vi "InitGen.vi"(4 "Offset":dbl format="%.4f", 5 "Gain":dbl=1.0 format="%.4f", 6 "Ext/nViTrig":bool, 7 "Waveform Data Array":dbl[](array[numeric]) format="%.4f", 8 "error in (no error)":errorcluster, 9 "Wave Per Pixel":i32, 10 "Sample Rate (Samp/s)":dbl=40000000.0 format="%.2f", 11 "FGEN Resource Name":refnum<k15>) -> (0 "error out":errorcluster, 2 "Actual Sample Rate":dbl, 3 "reference out":refnum<k15>)   [LabVIEW 2020]
uses:
  <instrlib>/niFgen/niFgen.llb/niFgen Output Mode.ctl
  <instrlib>/niFgen/niFgen.llb/niFgen_ctl Sample Clock Source Values (Ring).ctl
  <instrlib>/niFgen/niFgen.llb/niFgen Trigger Mode.ctl
  <instrlib>/niFgen/niFgen.llb/niFgen_ctl Trigger Source Values (Ring).ctl
  <instrlib>/niFgen/niFgen.llb/niFgen_ctl Exported Signal Desination Values (ComboBox).ctl
  <instrlib>/niFgen/niFgen.llb/niFgen_ctl Exported Signal Name Values (Ring).ctl
  <instrlib>/niFgen/niFgen.llb/niFgen Create Waveform (DBL).vi
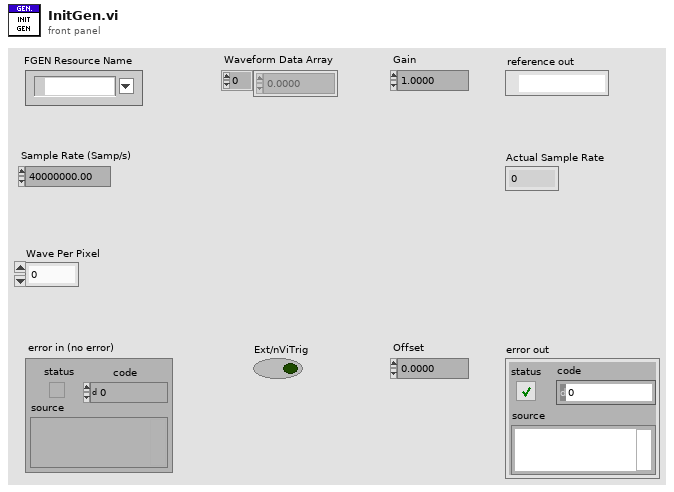
[diagram p1: front panel]
types:
  T1 = typedef "niFgen_ctl Exported Signal Name Values (Ring).ctl" = u16
  T2 = typedef "niFgen_ctl Exported Signal Desination Values (ComboBox).ctl" = string
  T3 = typedef "niFgen_ctl Trigger Source Values (Ring).ctl" = string
  T4 = typedef "niFgen Trigger Mode.ctl" = i32
  T5 = typedef "niFgen_ctl Sample Clock Source Values (Ring).ctl" = string
  T6 = typedef "niFgen Output Mode.ctl" = u32
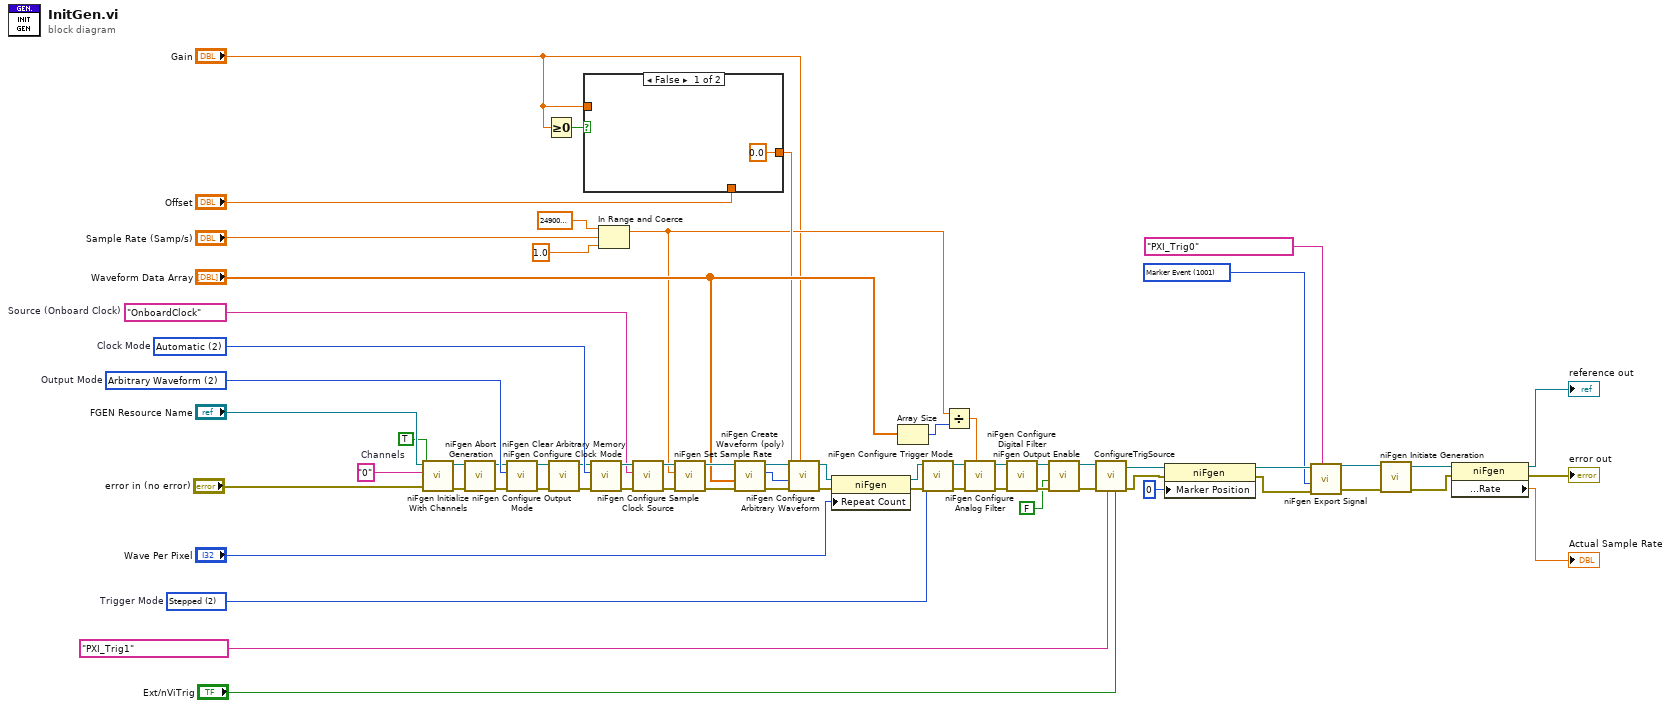
[diagram p0: block diagram]
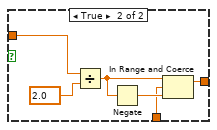
[diagram p2: hidden frame]
diagram:
  w1 = T1 1001 items=["Sample Clock"=101, "Sample Clock Timebase"=1006, "Reference Clock"=102, "Onboard Reference Clock"=1019, "Start Trigger"=1004, "Script Trigger"=103, "Marker Event"=1001, "Data Marker Event"=108, "Ready For Start Event"=105, "Started Event"=106, "Done Event"=107, "Synchronization Pulse"=1007, "Sync Out"=1002] ("Signal")
  w30 = T4 2 items=["Single", "Continuous", "Stepped", "Burst"]  # Trigger Mode
  w50 = T5 "OnboardClock"  # Source (Onboard Clock)
  w64 = u32 2 items=["Hi Resolution Sampling", "Divide Down Sampling", "Automatic"]  # Clock Mode
  w59 = T6 2 items=["Standard Function", "Frequency List", "Arbitrary Waveform", "Arbitrary Sequence", "Script"]  # Output Mode
  w66 = "0"  # Channels
  n1 = call <instrlib>:"niFgen Initialize With Channels.vi"("error in (no error)"="error in (no error)", "Reset Device (default: True)"=TRUE, "Channel Name"=w66, "Resource Name"="FGEN Resource Name") -> ("error out"=w55:errorcluster, "Instrument Handle Out"=w56:refnum<k15>)  [unwired: 6 in]
  n2 = call <instrlib>:"niFgen Abort Generation.vi"("error in (no error)"=w55, "Instrument Handle"=w56) -> ("error out"=w57:errorcluster, "Instrument Handle Out"=w58:refnum<k15>)  [unwired: 8 in]
  n3 = call <instrlib>:"niFgen Configure Output Mode.vi"("error in (no error)"=w57, "Output Mode (default: 0=Standard Function)"=w59, "Instrument Handle"=w58) -> ("error out"=w63:errorcluster, "Instrument Handle Out"=w60:refnum<k15>)  [unwired: 6 in]
  n4 = Greater Or Equal To 0?(x="Gain") -> (x >= 0?=w13:bool)
  n5 = call <instrlib>:"niFgen Clear Arbitrary Memory.vi"("error in (no error)"=w63, "Instrument Handle"=w60) -> ("error out"=w62:errorcluster, "Instrument Handle Out"=w61:refnum<k15>)  [unwired: 8 in]
  n6 = case shown="False" w13 {
    tunnel: "Gain" -> [_ w70]
    tunnel: "Offset" -> [_ w69]
    tunnel: [0.0 ("Offset") w68] -> w28
    frame False {
    }
    frame True {
      n7 = Divide(x=w70, y=2.0) -> (x/y=w72:dbl)
      n8 = Negate(x=w72) -> (-x=w71:dbl)
      n9 = In Range and Coerce(upper limit=w72, x=w69, lower limit=w71) -> (coerced(x)=w68:dbl)  [unwired: 1 out]
    }
  }
  n10 = call <instrlib>:"niFgen Configure Clock Mode.vi"("error in (no error)"=w62, "Clock Mode (default: 1=divide down)"=w64, "Instrument Handle"=w61) -> ("error out"=w51:errorcluster, "Instrument Handle Out"=w52:refnum<k15>)  [unwired: 7 in]
  n11 = In Range and Coerce(upper limit=249000000.0, x="Sample Rate (Samp/s)", lower limit=1.0) -> (coerced(x)=w23:dbl)  [unwired: 1 out]
  n12 = call <instrlib>:"niFgen Configure Sample Clock Source.vi"("error in (no error)"=w51, "Source (Onboard Clock)"=w50, "Instrument Handle"=w52) -> ("error out"=w54:errorcluster, "Instrument Handle Out"=w53:refnum<k15>)  [unwired: 7 in]
  n13 = call <instrlib>:"niFgen Set Sample Rate.vi"("error in (no error)"=w54, "Sample Rate (Samp/s)"=w23, "Instrument Handle"=w53) -> ("error out"=w48:errorcluster, "Instrument Handle Out"=w49:refnum<k15>)  [unwired: 7 in]
  n14 = call-poly <instrlib>:"niFgen Create Waveform (poly).vi"("error in (no error)"=w48, "Waveform Data Array"="Waveform Data Array", "Instrument Handle"=w49) -> ("error out"=w46:errorcluster, "Waveform Handle"=w45:i32, "Instrument Handle Out"=w47:refnum<k15>)  [unwired: 6 in]
  n15 = call <instrlib>:"niFgen Configure Arbitrary Waveform.vi"("Gain"="Gain", "Offset"=w28, "error in (no error)"=w46, "Waveform Handle"=w45, "Instrument Handle"=w47) -> ("error out"=w43:errorcluster, "Instrument Handle Out"=w44:refnum<k15>)  [unwired: 5 in]
  n16 = property class="niFgen"(reference=w44, error in=w43, "Repeat Count"="Wave Per Pixel") -> (reference out=w32:refnum<k15>, error out=w31:errorcluster)
  n17 = Array Size(array="Waveform Data Array") -> (size(s)=w35:i32)
  n18 = call <instrlib>:"niFgen Configure Trigger Mode.vi"("error in (no error)"=w31, "Trigger Mode (default: 1=continuous)"=w30, "Instrument Handle"=w32) -> ("error out"=w41:errorcluster, "Instrument Handle Out"=w40:refnum<k15>)  [unwired: 7 in]
  n19 = Divide(x=w23, y=w35) -> (x/y=w34:dbl)
  n20 = call <instrlib>:"niFgen Configure Analog Filter.vi"("Filter Correction Frequency"=w34, "error in (no error)"=w41, "Instrument Handle"=w40) -> ("error out"=w36:errorcluster, "Instrument Handle Out"=w37:refnum<k15>)  [unwired: 7 in]
  n21 = call <instrlib>:"niFgen Configure Digital Filter.vi"("error in (no error)"=w36, "Instrument Handle"=w37) -> ("error out"=w39:errorcluster, "Instrument Handle Out"=w38:refnum<k15>)  [unwired: 8 in]
  n22 = call <instrlib>:"niFgen Output Enable.vi"("error in (no error)"=w39, "Output Enable (default: True)"=FALSE, "Instrument Handle"=w38) -> ("error out"=w14:errorcluster, "Instrument Handle Out"=w15:refnum<k15>)  [unwired: 7 in]
  n23 = call "ConfigureTrigSource.vi"("Ext/nViTrig"="Ext/nViTrig", "Source"=T3 "PXI_Trig1", "error in (no error)"=w14, "Instrument Handle"=w15) -> ("error out"=w7:errorcluster, "Instrument Handle Out"=w8:refnum<k15>)  [unwired: 6 in]
  n24 = property class="niFgen"(reference=w8, error in=w7, "Marker Position"=0 ("Arbitrary Waveform:Arbitrary Waveform Mode:Marker Position")) -> (reference out=w6:refnum<k15>, error out=w5:errorcluster)
  n25 = call <instrlib>:"niFgen Export Signal.vi"("Output Terminal (do not export)"=T2 "PXI_Trig0", "error in (no error)"=w5, "Signal"=w1, "Instrument Handle"=w6) -> ("error out"=w3:errorcluster, "Instrument Handle Out"=w4:refnum<k15>)  [unwired: 6 in]
  n26 = call <instrlib>:"niFgen Initiate Generation.vi"("error in (no error)"=w3, "Instrument Handle"=w4) -> ("error out"=w25:errorcluster, "Instrument Handle Out"=w26:refnum<k15>)  [unwired: 8 in]
  n27 = property class="niFgen"(reference=w26, error in=w25) -> (reference out=→"reference out":refnum<k15>, error out=→"error out":errorcluster, "Clocks:Sample Clock:Rate"=→"Actual Sample Rate":dbl)
